vi "Log Kommandos.vi"(9 "Init":bool, 11 "Kommandos":string) -> (3 "Kommandos out":string)   [LabVIEW 2020, in "Linearisierung v2.lvlib" / "Gasteiler.lvlib" / "HovaCAL_Interface.lvlib" / "Kommunikation.lvlib"]
uses:
  Kommunikation.lvlib
  Allgemein/allgemeine Sub-VIs.lvlib
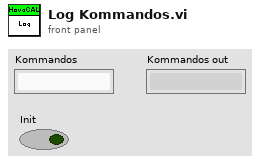
[diagram p1: front panel]
types:
  T1 = enum16{"open", "replace", "create", "open or create", "replace or create", "replace or create with confirmation"}
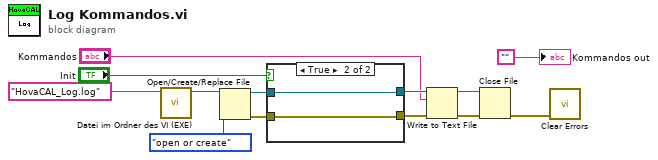
[diagram p0: block diagram]
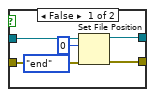
[diagram p2: hidden frame]
diagram:
  n1 = call "Datei im Ordner des VI (EXE).vi"("Dateiname"="HovaCAL_Log.log") -> ("Dateipfad im Ordner des Haupt-VIs"=w12:path)  [unwired: 8 in, 2 out]
  n2 = Open/Create/Replace File(file path (use dialog)=w12, operation (0:open)=T1."open or create" ("Operation (0:open)")) -> (refnum out=w11:refnum<file>, error out=w13:errorcluster)  [unwired: 4 in, 1 out]
  n3 = case shown="True" "Init" {
    tunnel: w13 -> [w19 w20]
    tunnel: w11 -> [w18 w21]
    tunnel: [w15 w21] -> w7
    tunnel: [w14 w20] -> w5
    frame False {
      n4 = Set File Position(offset (in bytes) (0)=i64 0 ("Offset (in Byte) (0)"), refnum=w18, from (0:start)=enum16{"start", "end", "current"}."end" ("Von (0:Start)"), error in=w19) -> (refnum out=w15:refnum<file>, error out=w14:errorcluster)
    }
    frame True {
    }
  }
  n5 = Write to Text File(file (use dialog)=w7, text="Kommandos", error in=w5) -> (refnum out=w6:refnum<file>, error out=w4:errorcluster)  [unwired: 1 in, 1 out]
  n6 = Close File(refnum=w6, error in=w4) -> (error out=w10:errorcluster)  [unwired: 1 out]
  n7 = call <vilib>:"Clear Errors.vi"("error in (no error)"=w10) -> ()  [unwired: 5 in, 2 out]
  "Kommandos out" <- ""
